vi "Send Dashboard Data.vi"   [LabVIEW 2012]
uses:
  BotStatus.vi
types:
  T1 = cluster{"Middle":bool, "InCannon":bool, "InFlipper":bool, "FlipperAtPlace":bool, "Bottom":bool, "FrisbeeDirection":bool}
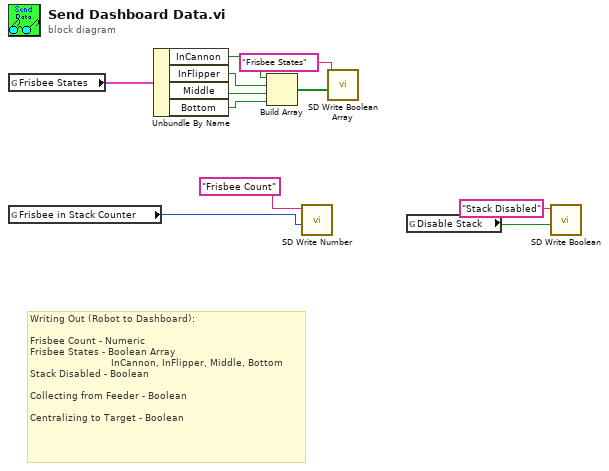
[diagram p0: block diagram]
diagram:
  # "Writing Out (Robot to Dashboard):\n\nFrisbee Count - Numeric\nFrisbee States - Boolean Array\n                           InCannon, InFlipper, Middle, Bottom\nStack Disabled - Boolean\n\nCollecting from Feeder - Boolean\n\nCentralizing to Target - Boolean"
  n1 = global read "BotStatus.vi" "Frisbee States"() -> (w9:T1)
  n2 = global read "BotStatus.vi" "Frisbee in Stack Counter"() -> (w11:i32)
  n3 = Unbundle By Name(w9) -> ("InCannon"=w8:bool, "InFlipper"=w7:bool, "Middle"=w6:bool, "Bottom"=w5:bool)
  n4 = Build Array(w8, w7, w6, w5) -> (w4:bool[])
  n5 = call <vilib>:"SD Write Number.vi"("Numeric"=w11, "Name"="Frisbee Count") -> ()  [unwired: 8 in, 2 out]
  n6 = call <vilib>:"SD Write Boolean Array.vi"("Boolean Array"=w4, "Name"="Frisbee States") -> ()  [unwired: 8 in, 2 out]
  n7 = global read "BotStatus.vi" "Disable Stack"() -> (w1:bool)
  n8 = call <vilib>:"SD Write Boolean.vi"("Boolean"=w1, "Name"="Stack Disabled") -> ()  [unwired: 8 in, 2 out]
